vi "RS232_Write-Read String 2.vi"(7 "Read Delay (ms)":u32=100, 9 "Write Buffer":string, 11 "Handle":u32) -> (1 "Bytes Read":u32, 3 "Read Buffer":string, 6 "Bytes Written":u32)   [LabVIEW 2018]
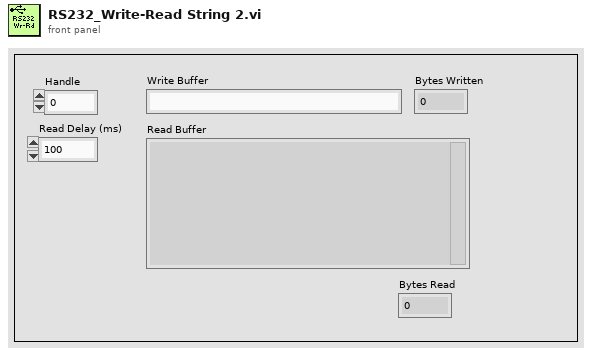
[diagram p1: front panel]
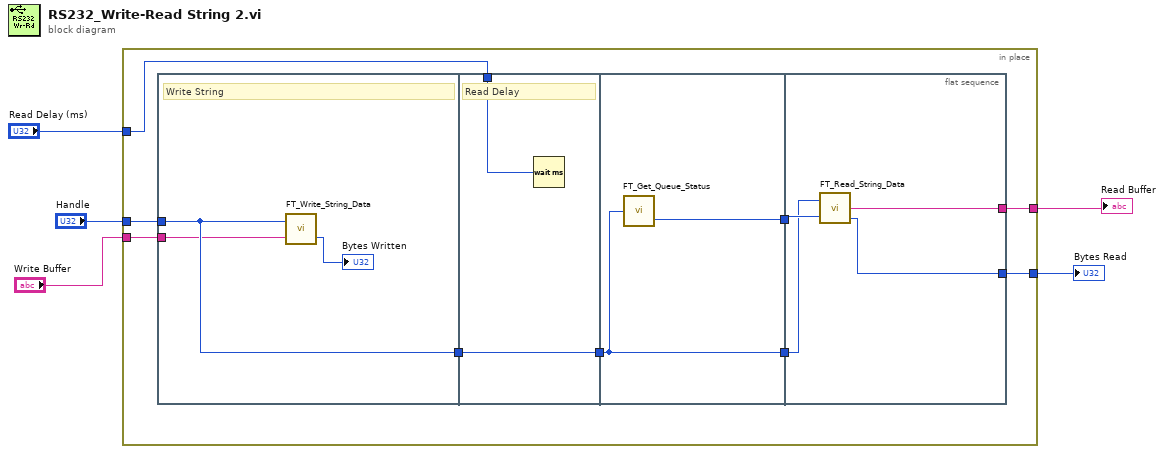
[diagram p0: block diagram]
diagram:
  n1 = in-place {
    in-place-border: "Handle" -> [w14]
    in-place-border: "Read Delay (ms)" -> [w13]
    in-place-border: [w8] -> w3
    in-place-border: [w7] -> w2
    in-place-border: "Write Buffer" -> [w6]
    n2 = flat-sequence {
      tunnel: w14 -> [w16]
      tunnel: [w16] -> w12
      tunnel: w6 -> [w15]
      tunnel: w13 -> [w19]
      tunnel: w12 -> [w18]
      tunnel: [w18] -> w11
      tunnel: w11 -> [w21]
      tunnel: [w21] -> w10
      tunnel: [w20] -> w9
      tunnel: w10 -> [w24]
      tunnel: w9 -> [w25]
      tunnel: [w23] -> w8
      tunnel: [w22] -> w7
      frame #0 {
        # "Write String"
        n3 = call "FT_Write_String_Data.vi"("Buffer"=w15, "Handle"=w16) -> ("Bytes Written"=→"Bytes Written":u32)  [unwired: 1 out]
      }
      frame #1 {
        # "Read Delay"
        n4 = Wait (ms)(milliseconds to wait=w19) -> ()  [unwired: 1 out]
      }
      frame #2 {
        n5 = call "FT_Get_Queue_Status.vi"("Handle"=w21) -> ("Bytes Waiting"=w20:u32)  [unwired: 1 out]
      }
      frame #3 {
        n6 = call "FT_Read_String_Data.vi"("Handle"=w24, "Bytes To Read"=w25) -> ("Read Data"=w23:string, "Bytes Read"=w22:u32)  [unwired: 1 out]
      }
    }
  }
  "Read Buffer" <- w3
  "Bytes Read" <- w2
